vi "Set State to Idle.vi"(8 "error in (no error)":errorcluster, 11 "Sequencer in":refnum<class "Sequencer.lvclass">) -> (0 "error out":errorcluster, 3 "Sequencer out":refnum<class "Sequencer.lvclass">)   [LabVIEW 2024, in "Ramses Sequencer.lvlib" / "Sequencer.lvclass"]
uses:
  Sequencer.lvclass
  typedef/Sequencer State -- enum.ctl
  Program Files (x86)/Enterative/Ramses Framework/Ramses Framework.lvlibp/Service/Service.lvclass
  C:/Program Files (x86)/Enterative/Ramses Framework/Ramses Framework.lvlibp/Service/Service.lvclass
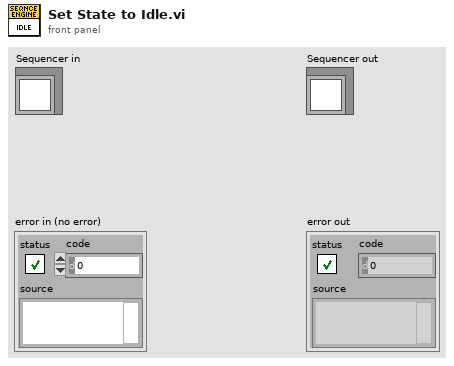
[diagram p1: front panel]
types:
  T1 = typedef "Ramses Sequencer.lvlib/Sequencer.lvclass/Sequencer State -- enum.ctl" = enum16{"Idle", "Running", "Paused", "Complete"}
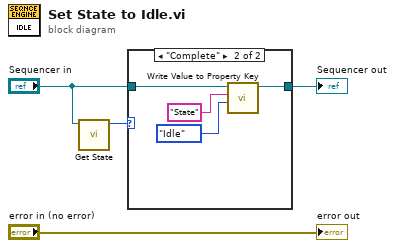
[diagram p0: block diagram]
diagram:
  n1 = call "Get State.vi"("Sequencer in"="Sequencer in") -> ("Sequencer State"=w1:T1)  [unwired: 9 in, 1 out]
  n2 = case shown="\"Complete\"" w1 {
    tunnel: [w5 w7] -> w3
    tunnel: "Sequencer in" -> [w5 w9]
    frame Default {
    }
    frame "Complete" {
      n3 = call "Write Value to Property Key.vi"("Value"=Sequencer_State_--_enum."Idle" ("Sequencer State"), "Key"="State", "Service in"=w9) -> ("Service out"=w7:refnum<class "Sequencer.lvclass">)  [unwired: 7 in, 1 out]
    }
  }
  "Sequencer out" <- w3
  "error out" <- "error in (no error)"
